vi "DestroyProtectedEvents.vi"(8 "error in (no error)":errorcluster, 11 "Measurement":refnum<class "Measurement.lvclass">) -> (0 "error out":errorcluster, 3 "Measurement out":refnum<class "Measurement.lvclass">)   [LabVIEW 2017, in "Measurement.lvclass"]
doc: "JKI State Machine Objects (SMO) 1.3.0.56\nJKI - JKI\nCopyright (c) 2017, JKI"
uses:
  Measurement.lvclass
  <vilib>/JKI/JKI SMO/SMO/SMO.lvclass
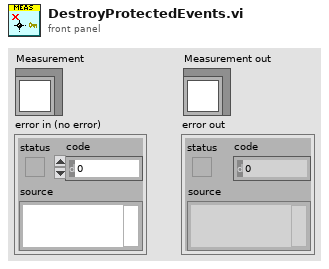
[diagram p1: front panel]
types:
  T1 = typedef "Measurement.lvclass/ProtectedEvents--Cluster.ctl" = cluster{"Initialize":refnum<user-event>}
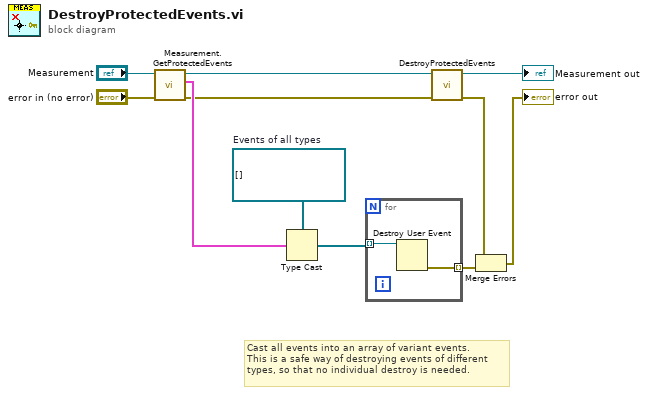
[diagram p0: block diagram]
diagram:
  w10 = refnum<user-event>[] []  # Events of all types
  # "Cast all events into an array of variant events.\nThis is a safe way of destroying events of different\ntypes, so that no individual destroy is needed."
  n1 = call "Measurement.GetProtectedEvents.vi"("error in (no error)"="error in (no error)", "Measurement in"="Measurement") -> ("error out"=w1:errorcluster, "Protected Events"=w2:T1, "Measurement out"=w3:refnum<class "Measurement.lvclass">)  [unwired: 7 in]
  n2 = Type Cast(type=w10, x=w2) -> (*(type *) &x=w8:refnum<user-event>[])
  n3 = for {
    tunnel: w8 -> [w13] mode=indexing
    tunnel: [w12] -> w9 mode=indexing
    n4 = Destroy User Event(user event=w13) -> (error out=w12:errorcluster)  [unwired: 1 in]
  }
  n5 = call-parent "DestroyProtectedEvents.vi"("error in (no error)"=w1, "SMO"=w3) -> ("error out"=w7:errorcluster, "SMO out"=→"Measurement out":refnum<class "Measurement.lvclass">)  [unwired: 8 in]
  n6 = Merge Errors(w7, w9) -> (→"error out":errorcluster)
